vi "VCI_ERR_INFO_CONVERT.vi"(1 "VCI_ERR_INFO":T2) -> (0 "VCI_ERR_INFO_1":T1)   [LabVIEW 2018, in "ControlCan.lvlib"]
uses:
  ControlCan.lvlib
  VCI_ERR_INFO.ctl
  VCI_ERR_INFO_1.ctl
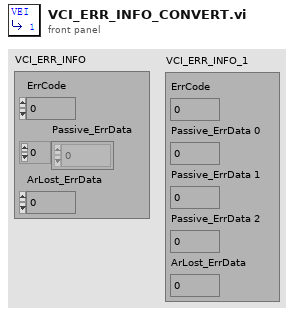
[diagram p1: front panel]
types:
  T1 = typedef "ControlCAN.lvlib/VCI_ERR_INFO_1.ctl" = cluster{"ErrCode":u32, "Passive_ErrData 0":u8, "Passive_ErrData 1":u8, "Passive_ErrData 2":u8, "ArLost_ErrData":u8}
  T2 = typedef "ControlCAN.lvlib/VCI_ERR_INFO.ctl" = cluster{"ErrCode":u32, "Passive_ErrData":u8[], "ArLost_ErrData":u8}
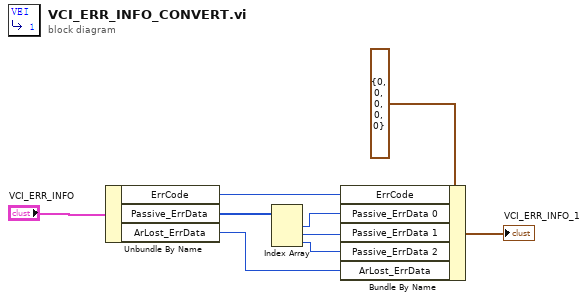
[diagram p0: block diagram]
diagram:
  n1 = Unbundle By Name("VCI_ERR_INFO") -> ("ErrCode"=w7:u32, "Passive_ErrData"=w6:u8[], "ArLost_ErrData"=w2:u8)
  n2 = Index Array(array=w6) -> (element #1=w5:u8, element #2=w4:u8, element #3=w3:u8)  [unwired: 3 in]
  n3 = Bundle By Name(cluster=T1 {"ErrCode"=0, "Passive_ErrData 0"=0, "Passive_ErrData 1"=0, "Passive_ErrData 2"=0, "ArLost_ErrData"=0} ("VCI_ERR_INFO_1"), "ErrCode"=w7, "Passive_ErrData 0"=w5, "Passive_ErrData 1"=w4, "Passive_ErrData 2"=w3, "ArLost_ErrData"=w2) -> (→"VCI_ERR_INFO_1":T1)
